vi "TimeBasedOutput.vi"() -> ()   [LabVIEW 2021]
panel:
  out "error out":errorcluster
  out "Output":dbl
  in  "Lookup table":cluster{"Hour":i32, "Output":dbl}[](array[cluster])=[{"Hour"=0, "Output"=0.0}, {"Hour"=12, "Output"=50.0}, {"Hour"=24, "Output"=0.0}]
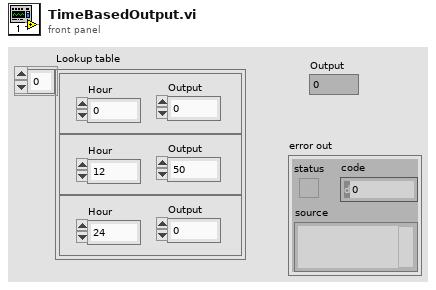
[diagram p1: front panel]
types:
  T1 = cluster{"second":i32, "minute":i32, "hour":i32, "day of month":i32, "month":i32, "year":i32, "day of week":i32, "day of year":i32, "is DST":i32}
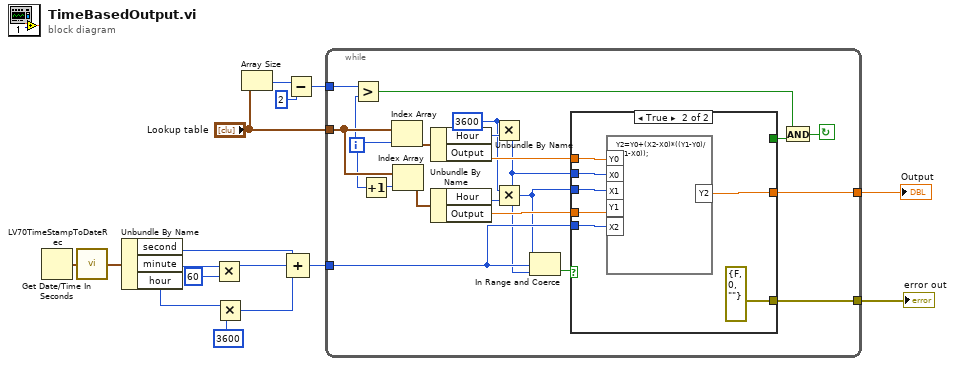
[diagram p0: block diagram]
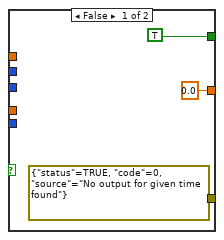
[diagram p2: hidden frame]
diagram:
  n1 = Get Date/Time In Seconds() -> (seconds since 1Jan1904=w1:timestamp)
  n2 = call <vilib>:"LV70TimeStampToDateRec.vi"("time stamp"=w1) -> ("date time rec"=w16:T1)
  n3 = Unbundle By Name(w16) -> ("second"=w9:i32, "minute"=w13:i32, "hour"=w15:i32)
  n4 = Multiply(x=w13, y=60) -> (x*y=w10:i32)
  n5 = Multiply(x=w15, y=3600) -> (x*y=w11:i32)
  n6 = Array Size(array="Lookup table") -> (size(s)=w5:i32)
  n7 = Subtract(x=w5, y=2) -> (x-y=w3:i32)
  n8 = Compound Arithmetic op=ADD(w9, w10, w11) -> (w8:i32)
  n9 = while {
    tunnel: "Lookup table" -> [w36]
    tunnel: w8 -> [w29]
    tunnel: [w28] -> w7
    tunnel: w3 -> [w27]
    tunnel: [w22] -> w2
    i -> [w26]
    stop <- w25 continue-if-true
    w18 = 3600 ("x")
    n10 = Greater?(x=w27, y=w26) -> (0:w24:bool)
    n11 = Increment(x=w26) -> (x+1=w35:i32)
    n12 = Index Array(array=w36, index=w26) -> (element=w34:cluster{"Hour":i32, "Output":dbl})
    n13 = Index Array(array=w36, index=w35) -> (element=w33:cluster{"Hour":i32, "Output":dbl})
    n14 = Unbundle By Name(w34) -> ("Hour"=w21:i32, "Output"=w31:dbl)
    n15 = Unbundle By Name(w33) -> ("Hour"=w19:i32, "Output"=w30:dbl)
    n16 = Multiply(x=w18, y=w21) -> (x*y=w20:i32)
    n17 = Multiply(x=w18, y=w19) -> (x*y=w17:i32)
    n18 = In Range and Coerce(upper limit=w17, x=w29, lower limit=w20) -> (In Range?=w32:bool)  [unwired: 1 out]
    n19 = case shown="True" w32 {
      tunnel: w20 -> [_ w46]
      tunnel: w31 -> [_ w45]
      tunnel: w17 -> [_ w44]
      tunnel: w30 -> [_ w43]
      tunnel: w29 -> [_ w42]
      tunnel: [0.0 ("Y2") w41] -> w28
      tunnel: [TRUE _] -> w23
      tunnel: [errorcluster {"status"=TRUE, "code"=0, "source"="No output for given time found"} ("error out") errorcluster {"status"=FALSE, "code"=0, "source"=""} ("error out")] -> w22
      frame False {
      }
      frame True {
        n20 = formula code="Y2=Y0+(X2-X0)*((Y1-Y0)/(X1-X0));"("Y0"=w45, "X0"=w46, "Y1"=w43, "X1"=w44, "X2"=w42) -> ("Y2"=w41:dbl)
      }
    }
    n21 = And(x=w24, y=w23) -> (x .and. y?=w25:bool)
  }
  "Output" <- w7
  "error out" <- w2
